vi "Pressure_Multiplexer_Server_Sub.vi"(0 "Single Pres Multiplexer":T2) -> (1 "Data Cluster":T1, 2 "DAQ Error":errorcluster)   [LabVIEW 2020]
uses:
  Device ID port info.ctl
  Controls/Fixed sampling rate Data Cluster.ctl
  <vilib>/Instr/_visa.llb/VISA Find Search Mode.ctl
  Ctls/Cmd list.ctl
  Pressure_Multiplexer_Server_Global.vi
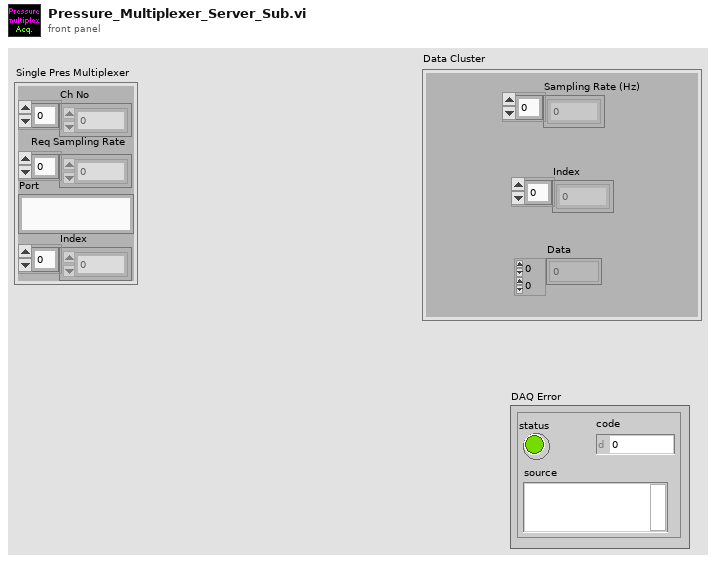
[diagram p1: front panel]
types:
  T1 = typedef "Fixed sampling rate Data Cluster.ctl" = cluster{"Sampling Rate (Hz)":dbl[], "Data":dbl[][], "Index":i32[]}
  T2 = typedef "Device ID port info.ctl" = cluster{"Ch No":i16[], "Req Sampling Rate":dbl[], "Port":string, "Index":i32[]}
  T3 = typedef "Trigger_Mode.ctl" = enum16{"Free Running", "Start on Trigger", "Trigger Every Block", "Trigger Every Sample"}
  T4 = typedef "Setup.ctl" = enum16{"Run Program", "Show Setup", "Save Current Setup", "Setup Front Panel"}
  T5 = typedef "Cmd list.ctl" = string
  T6 = typedef "VISA Find Search Mode.ctl" = u32
  T7 = typedef "Data values, Mode 0 (for datalog).ctl" = cluster{"Time Stamp":timestamp, "dt (us)":sgl, "dt_warn":u8, "Pressures":sgl[], "Statuses":u8[]}
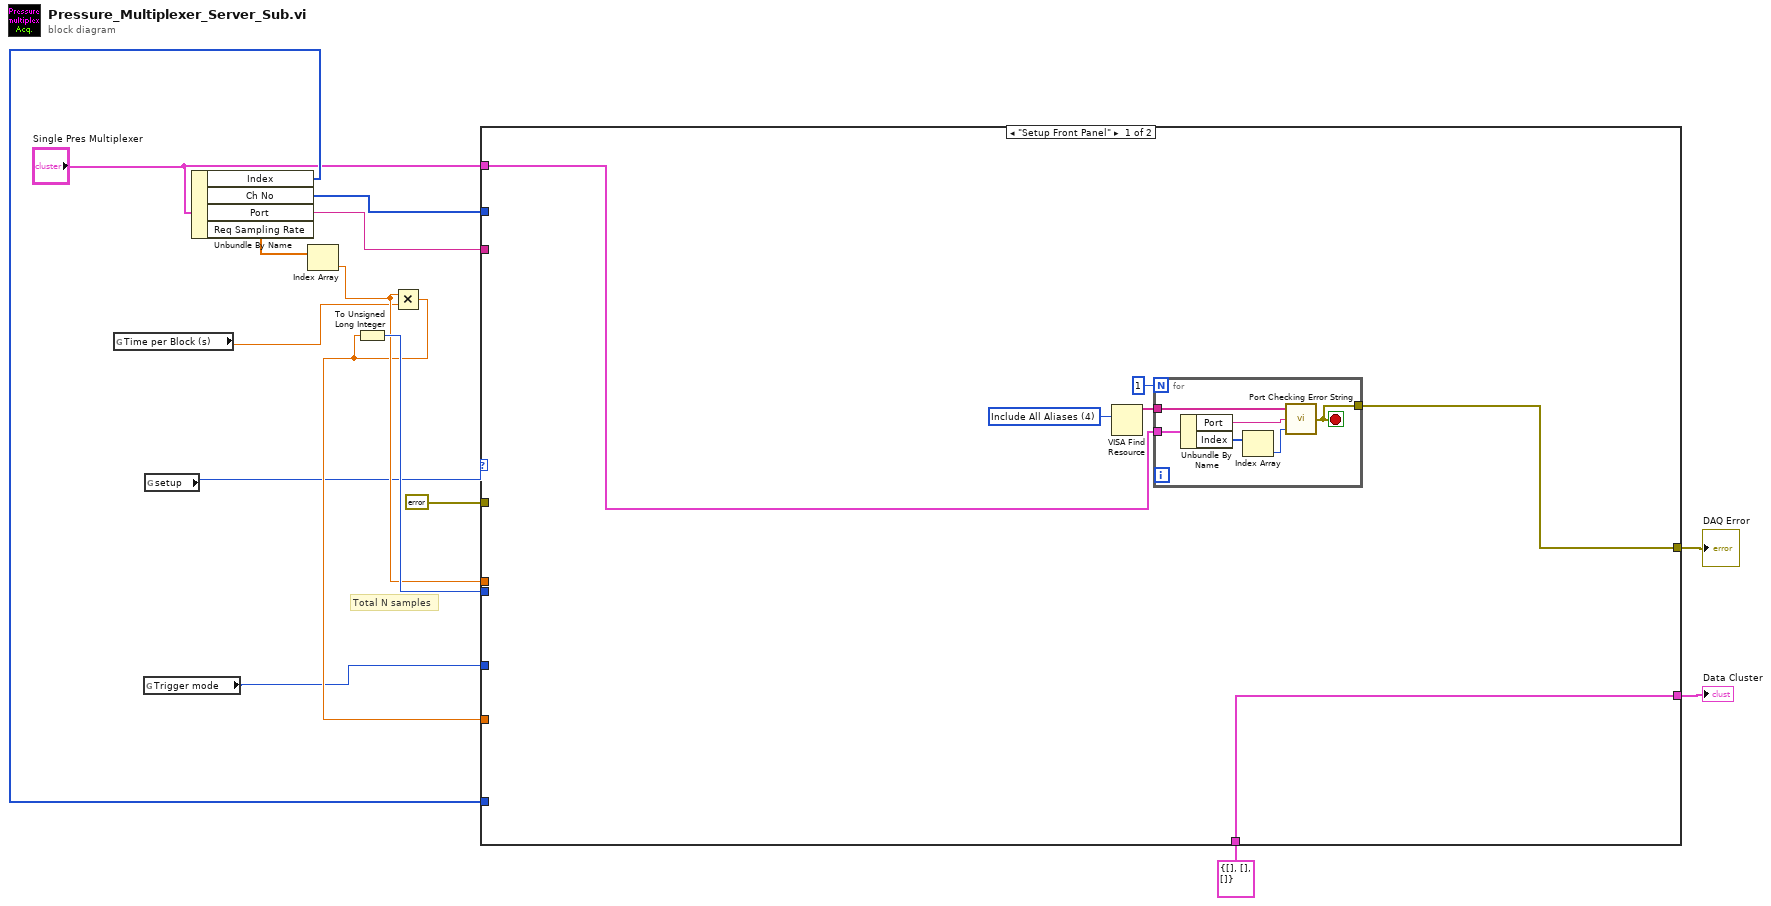
[diagram p0: block diagram]
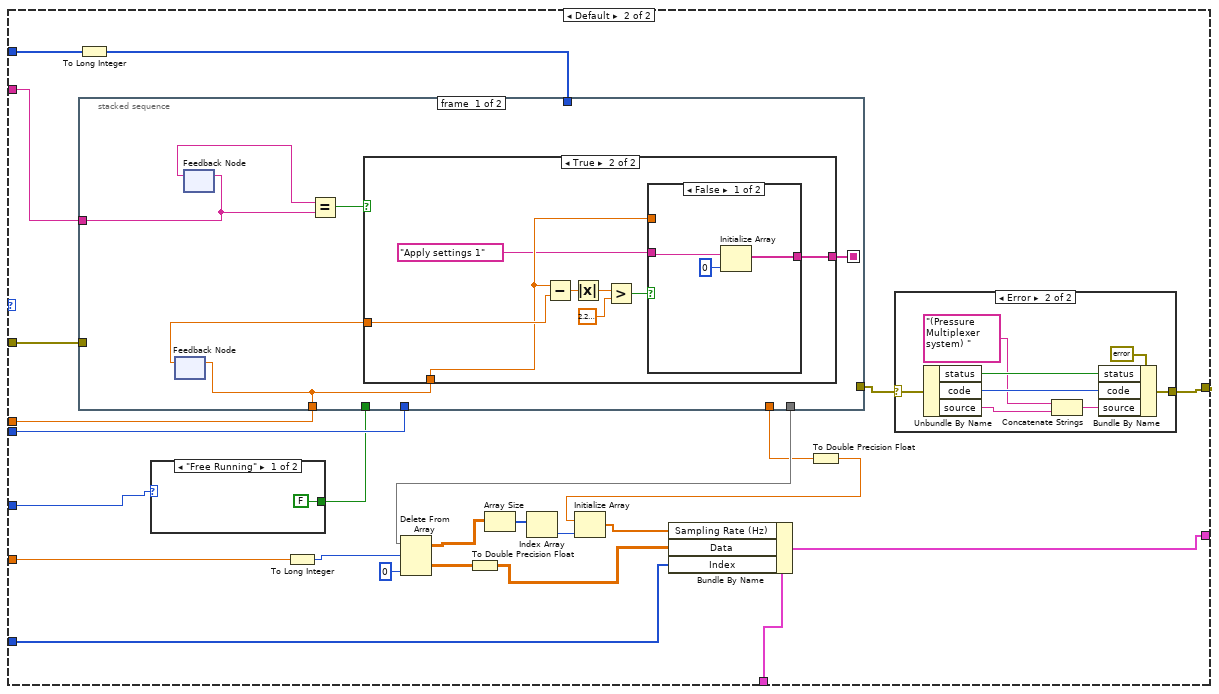
[diagram p2: hidden frame]
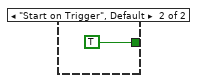
[diagram p3: hidden frame]
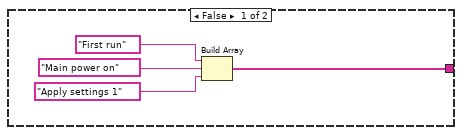
[diagram p4: hidden frame]
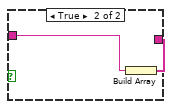
[diagram p5: hidden frame]
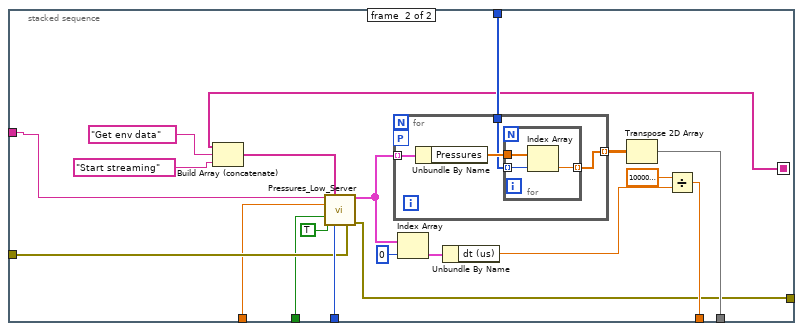
[diagram p6: hidden frame]
diagram:
  # "Total N samples"
  n1 = global read "Pressure_Multiplexer_Server_Global.vi" "Time per Block (s)"() -> (w3:dbl)
  n2 = global read "Pressure_Multiplexer_Server_Global.vi" "Trigger mode"() -> (w1:T3)
  n3 = global read "Pressure_Multiplexer_Server_Global.vi" "setup"() -> (w2:T4)
  n4 = Unbundle By Name("Single Pres Multiplexer") -> ("Index"=w9:i32[], "Ch No"=w8:i16[], "Port"=w11:string, "Req Sampling Rate"=w10:dbl[])
  n5 = Index Array(array=w10) -> (element=w12:dbl)  [unwired: 1 in]
  n6 = Multiply(x=w12, y=w3) -> (x*y=w6:dbl)
  n7 = To Unsigned Long Integer(number=w6) -> (unsigned 32bit integer=w14:u32)
  n8 = case shown="\"Setup Front Panel\"" w2 {
    tunnel: [w17 w52] -> w15
    tunnel: w14 -> [_ w51]
    tunnel: errorcluster {"status"=FALSE, "code"=0, "source"=""} ("Error in") -> [_ w48]
    tunnel: w6 -> [_ w47]
    tunnel: w12 -> [_ w35]
    tunnel: w11 -> [_ w36]
    tunnel: w8 -> [_ w46]
    tunnel: w9 -> [_ w33]
    tunnel: "Single Pres Multiplexer" -> [w19 _]
    tunnel: T1 {"Sampling Rate (Hz)"=[], "Data"=[], "Index"=[]} ("Data Cluster") -> [w16 w30]
    tunnel: [w16 w29] -> w4
    tunnel: w1 -> [_ w28]
    frame "Setup Front Panel" {
      w20 = T6 4 items=["Canonical Names Only"=0, "Aliases Only"=1, "Include Matching Aliases"=2, "Include All Aliases"=4] ("Search Mode")
      n9 = VISA Find Resource(10:w20) -> (3:w21:string[])  [unwired: 2 in, 2 out]
      n10 = for {
        N: 1 -> [_]
        tunnel: w19 -> [w27]
        tunnel: w21 -> [w23]
        tunnel: [w22] -> w17
        stop <- w22 stop-if-true
        n11 = Unbundle By Name(w27) -> ("Port"=w24:string, "Index"=w26:i32[])
        n12 = Index Array(array=w26) -> (element=w25:i32)  [unwired: 1 in]
        n13 = call "Port Checking Error String.vi"("Ch Index"=w25, "Port"=w24, "Available Ports"=w23) -> ("error out"=w22:errorcluster)  [unwired: 1 in]
      }
    }
    frame Default {
      n14 = To Long Integer(number=w46) -> (32bit integer=w37:i32[])
      n15 = case shown="\"Free Running\"" w28 {
        tunnel: [FALSE ("Wait for HW trigger") TRUE ("Wait for HW trigger")] -> w34
        frame "Free Running" {
        }
        frame "Start on Trigger", Default {
        }
      }
      n16 = stacked-sequence {
        seq-local: [w56 _] -> [_ w83]
        tunnel: w48 -> [_ w80]
        tunnel: w36 -> [w59 w81]
        tunnel: w35 -> [w55 w79]
        tunnel: [_ w88] -> w38
        tunnel: [_ w91] -> w49
        tunnel: [_ w97] -> w39
        tunnel: w51 -> [_ w87]
        tunnel: w37 -> [_ w86]
        tunnel: w34 -> [_ w78]
        frame #0 {
          n17 = feedback-in #1(w55) -> ()
          n18 = feedback #1() -> (w60:dbl)  [unwired: 1 in]
          n19 = feedback #2() -> (w58:string)  [unwired: 1 in]
          n20 = feedback-in #2(w59) -> ()
          n21 = Equal?(x=w58, y=w59) -> (x = y?=w57:bool)
          n22 = case shown="True" w57 {
            tunnel: w60 -> [_ w68]
            tunnel: w55 -> [_ w67]
            tunnel: [w61 w66] -> w56
            frame False {
              n23 = Build Array(T5 "First run" ("Command"), T5 "Main power on" ("Command"), T5 "Apply settings 1" ("Command")) -> (w61:T5[])
            }
            frame True {
              n24 = Subtract(x=w67, y=w68) -> (x-y=w70:dbl)
              n25 = Absolute Value(x=w70) -> (abs(x)=w71:dbl)
              n26 = Greater?(x=w71, y=2.220446049250313e-16) -> (0:w69:bool)
              n27 = case shown="False" w69 {
                tunnel: w67 -> [_ _]
                tunnel: [w73 w77] -> w66
                tunnel: T5 "Apply settings 1" ("Command") -> [w75 w76]
                frame False {
                  n28 = Initialize Array(w75, 0 ("dimension size")) -> (w73:T5[])
                }
                frame True {
                  n29 = Build Array(w76) -> (w77:T5[])
                }
              }
            }
          }
        }
        frame #1 {
          n30 = Build Array (concatenate)(w83, T5 "Get env data" ("Command"), T5 "Start streaming" ("Command")) -> (w82:T5[])
          n31 = call "Pressures_Low_Server.vi"("Serial port"=w81, "Commands"=w82, "Data rate (Hz)"=w79, "Wait for HW trigger"=w78, "Finite samples"=TRUE, "N samples"=w87, "Error in"=w80) -> ("P data (mode 0)"=w89:T7[], "Error out"=w88:errorcluster)  [unwired: 7 in]
          n32 = for {
            tunnel: [w99] -> w95 mode=indexing
            tunnel: w89 -> [w101] mode=indexing
            workers-P: _ -> [_]
            tunnel: w86 -> [w98]
            n33 = Unbundle By Name(w101) -> ("Pressures"=w100:sgl[])
            n34 = for {
              tunnel: w98 -> [w104] mode=indexing
              tunnel: w100 -> [w103]
              tunnel: [w102] -> w99 mode=indexing
              n35 = Index Array(array=w103, index=w104) -> (element=w102:sgl)
            }
          }
          n36 = Index Array(array=w89, index=0) -> (element=w93:T7)
          n37 = Unbundle By Name(w93) -> ("dt (us)"=w92:sgl)
          n38 = Transpose 2D Array(2D array=w95) -> (transposed array=w91:sgl[][])
          n39 = Divide(x=sgl 1000000.0 ("y"), y=w92) -> (x/y=w97:sgl)
        }
      }
      n40 = To Long Integer(number=w47) -> (32bit integer=w50:i32)
      n41 = Delete From Array(array=w49, length=w50, index (col)=0 ("disabled index (col)")) -> (deleted portion=w44:sgl[][], array with subset deleted=w43:sgl[][])  [unwired: 1 in]
      n42 = To Double Precision Float(number=w44) -> (double precision float=w32:dbl[][])
      n43 = Array Size(array=w43) -> (size(s)=w42:i32[])
      n44 = Index Array(array=w42) -> (element=w41:i32)  [unwired: 1 in]
      n45 = To Double Precision Float(number=w39) -> (double precision float=w45:dbl)
      n46 = Initialize Array(w45, w41) -> (w31:dbl[])
      n47 = Bundle By Name(cluster=w30, "Sampling Rate (Hz)"=w31, "Data"=w32, "Index"=w33) -> (w29:T1)
      n48 = case shown="Error" w38 {
        selector: w38 -> [w105 w106]
        tunnel: [w105 w113] -> w52
        frame No Error {
        }
        frame Error {
          n49 = Unbundle By Name(w106) -> ("status"=w111:bool, "code"=w110:i32, "source"=w109:string)
          n50 = Concatenate Strings("(Pressure Multiplexer system) " ("source"), w109) -> (w107:string)
          n51 = Bundle By Name(cluster=errorcluster {"status"=FALSE, "code"=0, "source"=""} ("DAQ Error"), "status"=w111, "code"=w110, "source"=w107) -> (w113:errorcluster)
        }
      }
    }
  }
  "DAQ Error" <- w15
  "Data Cluster" <- w4
